vi "Noise-Spectrum Level To Vrms.vi"(8 "Filtered Noise":dbl[](array[numeric]), 9 "dB Vrms of spectrum level = 0":dbl, 11 "Level In":T2) -> (1 "Max spectrum level":dbl, 3 "Level Out":T2)   [LabVIEW 2015]
uses:
  Controls/Level XCtl/Level Units.ctl
  <vilib>/Analysis/5stat.llb/RMS (DBL).vi
  PXI DAQ VIs/DAQ Engine VIs/PXI Globals.vi
  Utility VIs/Math VIs/Linear to dB (scalar).vi
  <vilib>/Analysis/NI_AALPro.lvlib
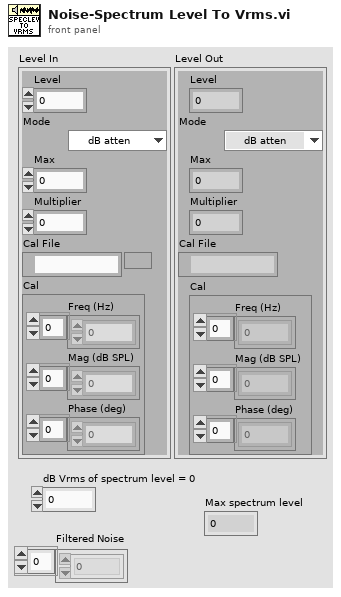
[diagram p1: front panel]
types:
  T1 = typedef "Level Units.ctl" = enum16{"dB atten", "dB SPL", "dB re 1 Vrms", "dB V/Hz½", "mW", "dB HL", "Volts", "dB mW"}
  T2 = cluster{"Level":dbl, "Mode":T1, "Max":dbl, "Multiplier":dbl, "Cal File":path, "Cal":cluster{"Freq (Hz)":dbl[], "Mag (dB SPL)":dbl[], "Phase (deg)":dbl[]}}
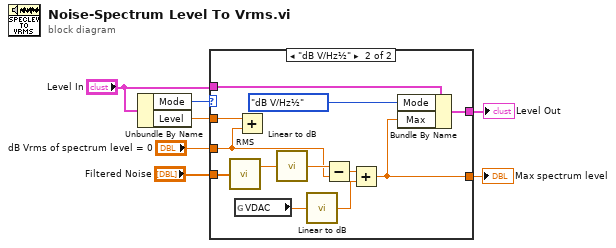
[diagram p0: block diagram]
diagram:
  n1 = Unbundle By Name("Level In") -> ("Mode"=w4:T1, "Level"=w6:dbl)
  n2 = case shown="\"dB V/Hz½\"" w4 {
    tunnel: "Level In" -> [w8 w20]
    tunnel: [w8 w17] -> w3
    tunnel: w6 -> [_ w18]
    tunnel: "dB Vrms of spectrum level = 0" -> [_ w13]
    tunnel: "Filtered Noise" -> [_ w16]
    tunnel: [_ w9] -> w1
    frame "dB atten", Default {
    }
    frame "dB V/Hz½" {
      n3 = call-poly <vilib>:"RMS.vi"("X"=w16) -> ("rms value"=w15:dbl)  [unwired: 1 out]
      n4 = global read "PXI Globals.vi" "VDAC"() -> (w11:dbl)
      n5 = Add(x=w18, y=w13) -> ()  [unwired: 1 out]
      n6 = call-poly "Linear to dB.vi"("Linear"=w15) -> ("dB"=w14:dbl)
      n7 = call-poly "Linear to dB.vi"("Linear"=w11) -> ("dB"=w10:dbl)
      n8 = Subtract(x=w14, y=w13) -> (x-y=w12:dbl)
      n9 = Add(x=w12, y=w10) -> (x+y=w9:dbl)
      n10 = Bundle By Name(cluster=w20, "Mode"=Level_Units."dB V/Hz½", "Max"=w9) -> (w17:T2)
    }
  }
  "Level Out" <- w3
  "Max spectrum level" <- w1
